vi "_get configuration data.vi"(8 "error in (no error)":errorcluster, 11 "refnum in":T1) -> (0 "error out":errorcluster, 3 "refnum out":T1)   [LabVIEW 2017]
uses:
  DSFConfig.lvlib
  DSF Config Data RefNum.ctl
  Controls/dsf configuration file/1.0.0/DSF Channel Info.ctl
  Controls/dsf configuration file/1.0.0/DSF Channel.ctl
  Controls/dsf configuration file/1.0.0/DSF Transfer Info.ctl
  Controls/dsf configuration file/1.0.0/DSF Transfer.ctl
  Controls/dsf configuration file/1.0.0/DSF Timing Info.ctl
  Controls/dsf configuration file/1.0.0/DSF Group Info.ctl
  Controls/dsf configuration file/1.0.0/DSF Group.ctl
  DSF Plugin Info.ctl
  Controls/dsf configuration file/1.0.0/DSF Plugin.ctl
  Controls/dsf configuration file/1.0.0/Version Info.ctl
  Controls/dsf configuration file/1.0.0/DSF Settings Info.ctl
  Controls/dsf configuration file/1.0.0/DSF Settings.ctl
  Controls/dsf configuration file/1.0.0/DSF Config.ctl
panel:
  out "dirty":bool
  out "path":path
  out "dsf configuration":T2
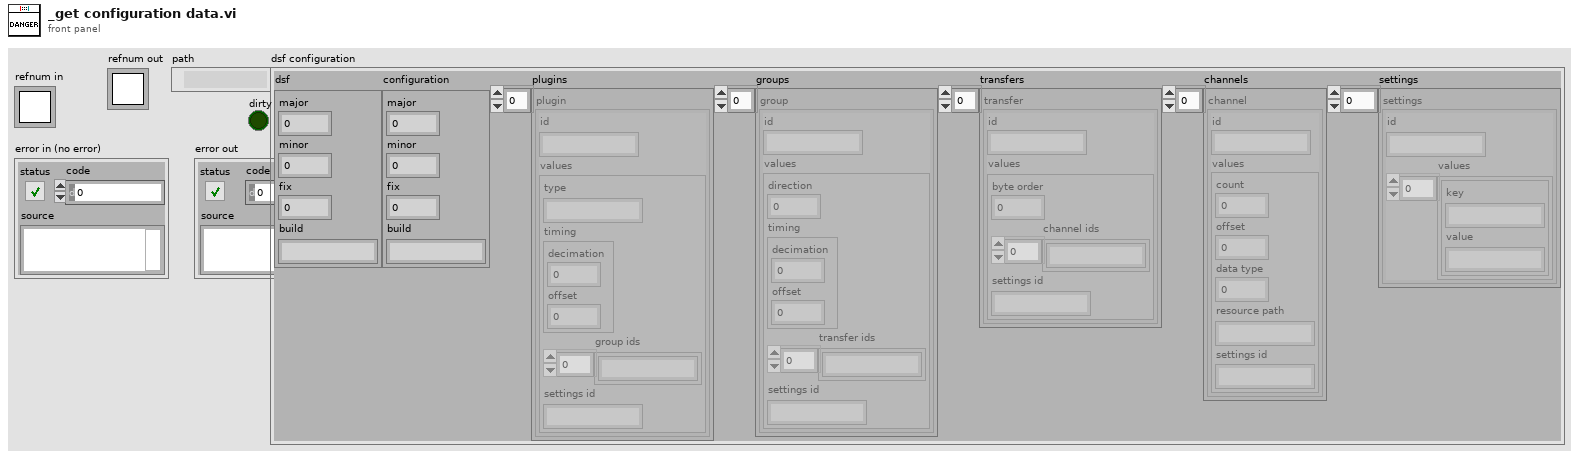
[diagram p1: front panel]
types:
  T1 = typedef "DSFConfig.lvlib/DSF Config Data RefNum.ctl" = refnum<k1>
  T2 = typedef "DSFConfig.lvlib/DSF Config.ctl" = cluster{"dsf":T3, "configuration":T3, "plugins":T4[], "groups":T7[], "transfers":T9[], "channels":T11[], "settings":T13[]}
  T3 = typedef "DSFConfig.lvlib/Version Info.ctl" = cluster{"major":u32, "minor":u32, "fix":u32, "build":string}
  T4 = typedef "DSFConfig.lvlib/DSF Plugin.ctl" = cluster{"id":string, "values":T5}
  T5 = typedef "DSFConfig.lvlib/DSF Plugin Info.ctl" = cluster{"type":string, "timing":T6, "group ids":string[], "settings id":string}
  T6 = typedef "DSFConfig.lvlib/DSF Timing Info.ctl" = cluster{"decimation":i32, "offset":i32}
  T7 = typedef "DSFConfig.lvlib/DSF Group.ctl" = cluster{"id":string, "values":T8}
  T8 = typedef "DSFConfig.lvlib/DSF Group Info.ctl" = cluster{"direction":i32, "timing":T6, "transfer ids":string[], "settings id":string}
  T9 = typedef "DSFConfig.lvlib/DSF Transfer.ctl" = cluster{"id":string, "values":T10}
  T10 = typedef "DSFConfig.lvlib/DSF Transfer Info.ctl" = cluster{"byte order":i32, "channel ids":string[], "settings id":string}
  T11 = typedef "DSFConfig.lvlib/DSF Channel.ctl" = cluster{"id":string, "values":T12}
  T12 = typedef "DSFConfig.lvlib/DSF Channel Info.ctl" = cluster{"count":i32, "offset":i32, "data type":i32, "resource path":string, "settings id":string}
  T13 = typedef "DSFConfig.lvlib/DSF Settings.ctl" = cluster{"id":string, "values":T14}
  T14 = typedef "DSFConfig.lvlib/DSF Settings Info.ctl" = cluster{"key":string, "value":string}[]
  T15 = typedef "DSFConfig.lvlib/Config Queue.ctl" = refnum<queue>
  T16 = typedef "DSFConfig.lvlib/Config Data.ctl" = cluster{"dsf configuration":T2, "path":path, "dirty":bool}
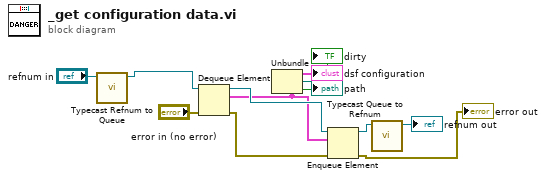
[diagram p0: block diagram]
diagram:
  n1 = call "Typecast Refnum to Queue.vi"("refnum in"="refnum in") -> ("queue out"=w11:T15)  [unwired: 10 in]
  n2 = Dequeue Element(queue=w11, error in (no error)="error in (no error)") -> (queue out=w5:T15, element=w1:T16, error out=w4:errorcluster)  [unwired: 1 in, 1 out]
  n3 = Unbundle(w1) -> ("dsf configuration"=→"dsf configuration":T2, "path"=→"path":path, "dirty"=→"dirty":bool)
  n4 = Enqueue Element(queue=w5, element=w1, error in (no error)=w4) -> (queue out=w6:T15, error out=→"error out":errorcluster)  [unwired: 2 out]
  n5 = call "Typecast Queue to Refnum.vi"("queue in"=w6) -> ("refnum out"=→"refnum out":T1)  [unwired: 10 out]
